vi "Mirror Holt State.vi"(8 "error in (no error)":errorcluster, 11 "1553 Component in":refnum<class "1553 Component.lvclass">) -> (0 "error out":errorcluster, 3 "1553 Component out":refnum<class "1553 Component.lvclass">)   [LabVIEW 2020, in "BCI-1553 API.lvlib" / "1553 Component.lvclass"]
doc: "Copies the current contents of the 1553 Session hardware for a single component to the component's Virtual Memory."
uses:
  1553 Component.lvclass
  1553 Component.lvclass/1553 Component.ctl
  Dependencies/FPGA Interface/FPGA Interface.lvclass
  Dependencies/Virtual Memory Unit/Virtual Memory Unit.lvclass
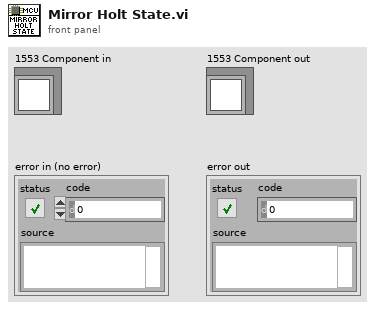
[diagram p1: front panel]
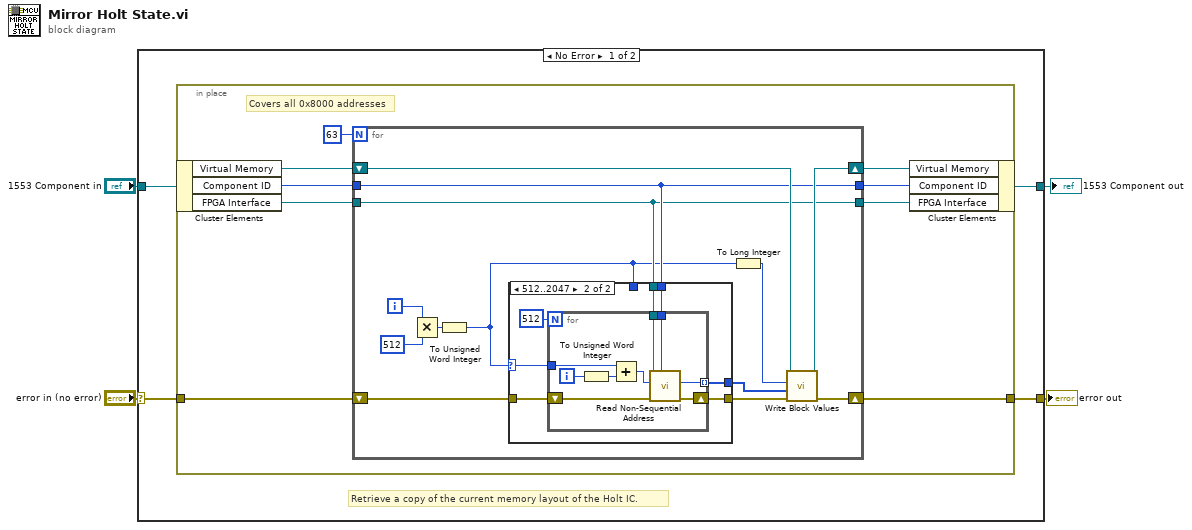
[diagram p0: block diagram]
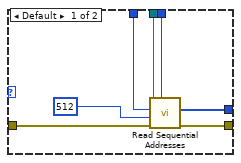
[diagram p2: hidden frame]
diagram:
  n1 = case shown="No Error" "error in (no error)" {
    selector: "error in (no error)" -> [w5 w54]
    tunnel: [w8 w55] -> w4
    tunnel: [w7 w54] -> w3
    tunnel: "1553 Component in" -> [w6 w55]
    frame No Error {
      # "Retrieve a copy of the current memory layout of the Holt IC."
      n2 = in-place {
        in-place-border: w5 -> [w17]
        in-place-border: [w16] -> w7
        # "Covers all 0x8000 addresses"
        n3 = in-place-cluster #1(w6) -> ("Virtual Memory"=w14:refnum<class "Virtual Memory Unit.lvclass">, "Component ID"=w13:u8, "FPGA Interface"=w12:refnum<class "FPGA Interface.lvclass">)
        n4 = for {
          N: 63 -> [_]
          tunnel: w12 -> [w21]
          tunnel: w13 -> [w22]
          shift-right: [w23] -> w11
          shift-left: w14 -> [w24]
          tunnel: [w22] -> w10
          tunnel: [w21] -> w9
          shift-right: [w25] -> w16
          shift-left: w17 -> [w30]
          i -> [w29]
          n5 = Multiply(x=w29, y=512) -> (x*y=w28:i32)
          n6 = To Unsigned Word Integer(number=w28) -> (unsigned 16bit integer=w18:u16)
          n7 = case shown="512..2047" w18 {
            selector: w18 -> [_ w38]
            tunnel: w30 -> [w37 w44]
            tunnel: w18 -> [w36 _]
            tunnel: [w35 w43] -> w26
            tunnel: w22 -> [w34 w41]
            tunnel: w21 -> [w33 w40]
            tunnel: [w32 w42] -> w20
            frame Default {
              n8 = call-dynamic "Read Sequential Addresses.vi"("Target IC (1-8)"=w34, "error in (no error)"=w37, "Addresses to Read"=u16 512 ("y"), "Starting Address"=w36, "FPGA Interface in"=w33) -> ("error out"=w35:errorcluster, "Data"=w32:u16[])  [unwired: 5 in]
            }
            frame 512..2047 {
              n9 = for {
                N: 512 -> [_]
                tunnel: [w51] -> w42 mode=indexing
                tunnel: w41 -> [w50]
                tunnel: w40 -> [w49]
                tunnel: w38 -> [w48]
                shift-right: [w52] -> w43
                shift-left: w44 -> [w53]
                i -> [w47]
                n10 = To Unsigned Word Integer(number=w47) -> (unsigned 16bit integer=w45:u16)
                n11 = Add(x=w48, y=w45) -> (x+y=w46:u16)
                n12 = call-dynamic "Read Non-Sequential Address.vi"("Target IC (1-8)"=w50, "error in (no error)"=w53, "Address"=w46, "FPGA Interface in"=w49) -> ("error out"=w52:errorcluster, "Data"=w51:u16)  [unwired: 6 in]
              }
            }
          }
          n13 = To Long Integer(number=w18) -> (32bit integer=w19:i32)
          n14 = call "Write Block Values.vi"("error in (no error)"=w26, "Write Block"=w20, "Start Index"=w19, "Virtual Memory Unit in"=w24) -> ("error out"=w25:errorcluster, "Virtual Memory Unit out"=w23:refnum<class "Virtual Memory Unit.lvclass">)  [unwired: 6 in]
        }
        n15 = in-place-cluster #1("Virtual Memory"=w11, "Component ID"=w10, "FPGA Interface"=w9) -> (w8:refnum<class "1553 Component.lvclass">)
      }
    }
    frame Error {
    }
  }
  "1553 Component out" <- w4
  "error out" <- w3
